vi "Druck nach Durchfluss Anpassen.vi"(10 "Sollwert Durchfluss":T2) -> (2 "Druck Ausgang":T1)   [LabVIEW 2020, in "Anlagengrenzwerte.lvlib"]
uses:
  Anlagengrenzwerte.lvlib
  Visualisierungs Elemente/Zahlen-Eingabefeld.ctl
  Visualisierungs Elemente/Zahlen-Ausgabefeld.ctl
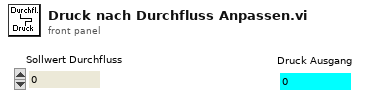
[diagram p1: front panel]
types:
  T1 = typedef "Zahlen-Ausgabefeld.ctl" = sgl
  T2 = typedef "Zahlen-Eingabefeld.ctl" = sgl
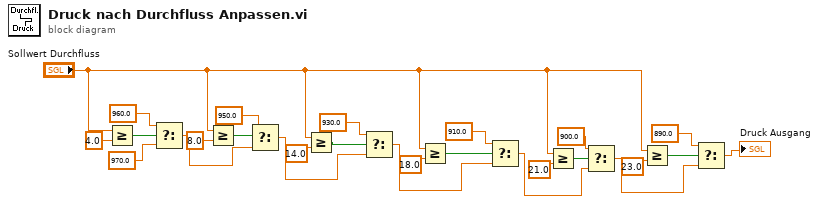
[diagram p0: block diagram]
diagram:
  n1 = Greater Or Equal?(x="Sollwert Durchfluss", y=T2 4.0) -> (x >= y?=w22:bool)
  n2 = Select(t=960.0 ("f"), s=w22, f=970.0) -> (s? t:f=w19:dbl)
  n3 = Greater Or Equal?(x="Sollwert Durchfluss", y=T2 8.0) -> (x >= y?=w25:bool)
  n4 = Select(t=950.0, s=w25, f=w19) -> (s? t:f=w15:dbl)
  n5 = Greater Or Equal?(x="Sollwert Durchfluss", y=T2 14.0) -> (x >= y?=w16:bool)
  n6 = Select(t=930.0 ("f"), s=w16, f=w15) -> (s? t:f=w11:dbl)
  n7 = Greater Or Equal?(x="Sollwert Durchfluss", y=T2 18.0) -> (x >= y?=w12:bool)
  n8 = Select(t=910.0 ("f"), s=w12, f=w11) -> (s? t:f=w3:dbl)
  n9 = Greater Or Equal?(x="Sollwert Durchfluss", y=T2 21.0) -> (x >= y?=w5:bool)
  n10 = Select(t=900.0 ("f"), s=w5, f=w3) -> (s? t:f=w2:dbl)
  n11 = Greater Or Equal?(x="Sollwert Durchfluss", y=T2 23.0) -> (x >= y?=w10:bool)
  n12 = Select(t=890.0 ("f"), s=w10, f=w2) -> (s? t:f=→"Druck Ausgang":dbl)
